vi "WPI_DMAAddChannelToStream_Encoder.vi"(7 "EncoderDevRef":T1={"DevStatus"={"status"=FALSE, "code"=0, "source"=""}, "EncoderIndex"=enum."Invalid", "CounterIndex"=enum."Invalid", "DistancePerCount"=1.0, "Decoding Type"=enum."4x"}, 8 "error in (no error)":errorcluster, 10 "Encoder Output Type":T5, 11 "DMARef":T6) -> (0 "error out":errorcluster, 3 "DMARef":T6)   [LabVIEW 2017]
doc: "Specifies the data transferred in the DMA stream. Wire a device reference from the other WPI Robotics Library Open VIs to specify the data you want to receive. The order that the AddChannel VIs add data to the DMA stream defines the order that the Read VI returns the data.\n\nSpecifies the encoder data transferred in the DMA stream.\n\nYou must open a reference to a DMA stream with the Open VI before using this VI.\n\nThis software is licensed. Open the labview\\readme\\WPI Robotics Library Open Source License.txt file for more information."
uses:
  <vilib>/Rock Robotics/WPI/DMA/WPI_DMARef.ctl
  <vilib>/Rock Robotics/WPI/DMA/WPI_DMAEncoderOutputType.ctl
  <vilib>/Rock Robotics/WPI/Encoder/WPI_EncoderDevRef.ctl
  <vilib>/Rock Robotics/SystemInterfaces/Encoder/FPGA_EncoderIdx.ctl
  <vilib>/Rock Robotics/SystemInterfaces/Counter/FPGA_CounterCtrSystemIndex.ctl
  <vilib>/Rock Robotics/WPI/Encoder/WPI_EncoderType.ctl
  <vilib>/Rock Robotics/WPI/DMA/WPI_DMAChannelTypeEnum.ctl
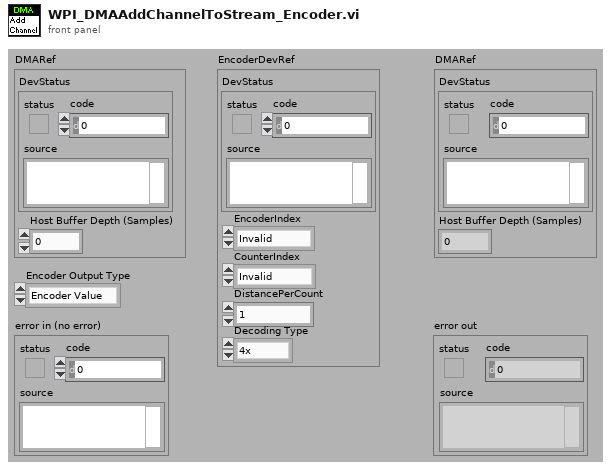
[diagram p1: front panel]
types:
  T1 = typedef "WPI_EncoderDevRef.ctl" = cluster{"DevStatus":errorcluster, "EncoderIndex":T2, "CounterIndex":T3, "DistancePerCount":dbl, "Decoding Type":T4}
  T2 = typedef "FPGA_EncoderIdx.ctl" = enum8{"Enc 0", "Enc 1", "Enc 2", "Enc 3", "Enc 4", "Enc 5", "Enc 6", "Enc 7", "Invalid"}
  T3 = typedef "FPGA_CounterCtrSystemIndex.ctl" = enum8{"Ctr 0", "Ctr 1", "Ctr 2", "Ctr 3", "Ctr 4", "Ctr 5", "Ctr 6", "Ctr 7", "Invalid"}
  T4 = typedef "WPI_EncoderType.ctl" = enum16{"1x", "2x", "4x"}
  T5 = typedef "WPI_DMAEncoderOutputType.ctl" = enum16{"Encoder Value", "Timer Value"}
  T6 = typedef "WPI_DMARef.ctl" = cluster{"DevStatus":errorcluster, "Host Buffer Depth (Samples)":u32}
  T7 = typedef "WPI_DMAChannelTypeEnum.ctl" = enum16{"AI (Raw)", "AI (Avg)", "Accumulator", "DI (Raw) Onboard", "DI (Filtered) Onboard", "DI (Raw) MXP", "DI (Filtered) MXP", "Analog Trigger", "Counter", "Counter (Timer)", "Encoder", "Encoder (Timer)", "Time Stamp"}
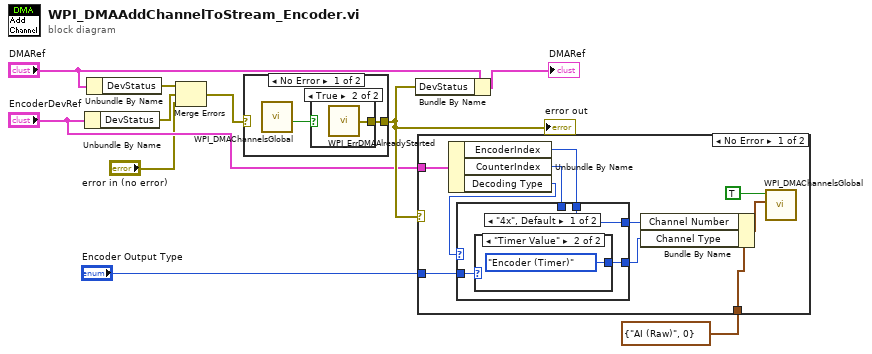
[diagram p0: block diagram]
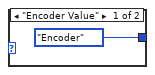
[diagram p2: hidden frame]
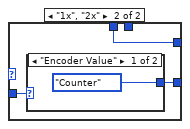
[diagram p3: hidden frame]
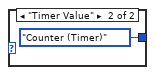
[diagram p4: hidden frame]
diagram:
  n1 = Unbundle By Name("EncoderDevRef") -> ("DevStatus"=w3:errorcluster)
  n2 = Unbundle By Name("DMARef") -> ("DevStatus"=w4:errorcluster)
  n3 = Merge Errors(w4, w3, "error in (no error)") -> (w1:errorcluster)
  n4 = case shown="No Error" w1 {
    selector: w1 -> [_ w14]
    tunnel: [w11 w14] -> w9
    frame No Error {
      n5 = call <vilib>:"WPI_DMAChannelsGlobal.vi"() -> ("Started"=w12:bool)  [unwired: 4 in, 7 out]
      n6 = case shown="True" w12 {
        tunnel: [_ w13] -> w11
        frame False {
        }
        frame True {
          n7 = call <vilib>:"WPI_ErrDMAAlreadyStarted.vi"() -> ("error out"=w13:errorcluster)
        }
      }
    }
    frame Error {
    }
  }
  "error out" <- w9
  n8 = Bundle By Name(cluster="DMARef", "DevStatus"=w9) -> (→"DMARef":T6)
  n9 = case shown="No Error" w9 {
    tunnel: "EncoderDevRef" -> [w23 _]
    tunnel: cluster{"Channel Type":T7, "Channel Number":u8} {"Channel Type"=enum."AI (Raw)", "Channel Number"=0} ("Channel") -> [w22 _]
    tunnel: "Encoder Output Type" -> [w19 _]
    frame No Error {
      n10 = Unbundle By Name(w23) -> ("EncoderIndex"=w17:T2, "CounterIndex"=w18:T3, "Decoding Type"=w16:T4)
      n11 = case shown="\"4x\", Default" w16 {
        tunnel: [w26 w32] -> w20
        tunnel: w19 -> [w27 w31]
        tunnel: w18 -> [_ w30]
        tunnel: w17 -> [w25 _]
        tunnel: [w25 w30] -> w15
        frame "4x", Default {
          n12 = case shown="\"Timer Value\"" w27 {
            tunnel: [WPI_DMAChannelTypeEnum."Encoder" ("Channel Type") WPI_DMAChannelTypeEnum."Encoder (Timer)" ("Channel Type")] -> w26
            frame "Encoder Value" {
            }
            frame "Timer Value" {
            }
          }
        }
        frame "1x", "2x" {
          n13 = case shown="\"Encoder Value\"" w31 {
            tunnel: [WPI_DMAChannelTypeEnum."Counter" ("Channel Type") WPI_DMAChannelTypeEnum."Counter (Timer)" ("Channel Type")] -> w32
            frame "Encoder Value" {
            }
            frame "Timer Value" {
            }
          }
        }
      }
      n14 = Bundle By Name(cluster=w22, "Channel Number"=w15, "Channel Type"=w20) -> (w21:cluster{"Channel Type":T7, "Channel Number":u8})
      n15 = call <vilib>:"WPI_DMAChannelsGlobal.vi"("Channel"=w21, "Add"=TRUE) -> ()  [unwired: 2 in, 8 out]
    }
    frame Error {
    }
  }
